vi "Log Interlock to the Caller.vi"(6 "Interlock in":refnum<class "Interlock.lvclass">, 8 "error in (no error)":errorcluster, 11 "CO2 Actor in":refnum<class "CO2 Actor.lvclass">) -> (0 "error out":errorcluster, 3 "CO2 Actor out":refnum<class "CO2 Actor.lvclass">)   [LabVIEW 2015, in "cRIO-Carbondioxide.lvlib" / "CO2-Actor.lvlib" / "CO2 Actor.lvclass"]
uses:
  CO2 Actor.lvclass
  Interlocks/Interlock/Interlock.lvclass
  Interlocks/Interlock/Interlock.lvclass/Interlock.ctl
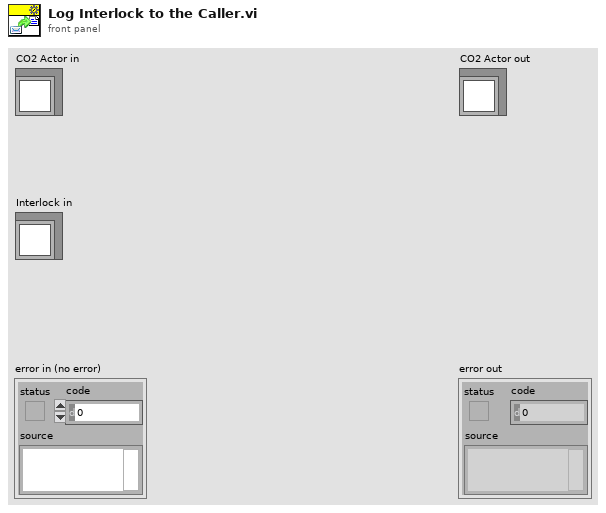
[diagram p1: front panel]
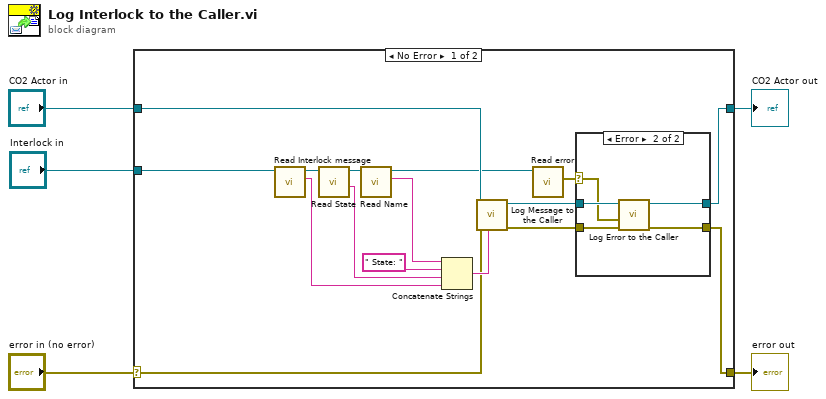
[diagram p0: block diagram]
diagram:
  n1 = case shown="No Error" "error in (no error)" {
    selector: "error in (no error)" -> [w13 w30]
    tunnel: [w6 w30] -> w4
    tunnel: [w8 w29] -> w2
    tunnel: "CO2 Actor in" -> [w15 w29]
    tunnel: "Interlock in" -> [w12 _]
    frame No Error {
      n2 = call "Read Interlock message.vi"("Interlock in"=w12) -> ("Interlock message"=w16:string, "Interlock out"=w17:refnum<class "Interlock.lvclass">)  [unwired: 9 in]
      n3 = call "Read State.vi"("Interlock in"=w17) -> ("State string"=w19:string, "Interlock out"=w21:refnum<class "Interlock.lvclass">)  [unwired: 8 in, 1 out]
      n4 = call "Read Name.vi"("Interlock in"=w21) -> ("Name"=w18:string, "Interlock out"=w11:refnum<class "Interlock.lvclass">)  [unwired: 9 in]
      n5 = Concatenate Strings(w18, " State: " ("string"), w19, w16) -> (w14:string)
      n6 = call-dynamic "Log Message to the Caller.vi"("String (\"\" = no message to send)"=w14, "error in (no error)"=w13, "CO2 Actor in"=w15) -> ("error out"=w7:errorcluster, "CO2 Actor out"=w9:refnum<class "CO2 Actor.lvclass">)  [unwired: 7 in]
      n7 = call "Read error.vi"("Interlock in"=w11) -> ("error"=w10:errorcluster)  [unwired: 9 in, 1 out]
      n8 = case shown="Error" w10 {
        selector: w10 -> [_ w24]
        tunnel: w7 -> [w22 w28]
        tunnel: w9 -> [w23 w27]
        tunnel: [w23 w26] -> w8
        tunnel: [w22 w25] -> w6
        frame No Error {
        }
        frame Error {
          n9 = call-dynamic "Log Error to the Caller.vi"("error in (no error)"=w28, "Error to log"=w24, "CO2 Actor in"=w27) -> ("error out"=w25:errorcluster, "CO2 Actor out"=w26:refnum<class "CO2 Actor.lvclass">)  [unwired: 7 in]
        }
      }
    }
    frame Error {
    }
  }
  "error out" <- w4
  "CO2 Actor out" <- w2
